vi "Increment Index.vi"(8 "error in (no error)":errorcluster, 11 "Abs_Waveform in":refnum<class "Abs_Waveform.lvclass">) -> (0 "error out":errorcluster, 3 "Abs_Waveform out":refnum<class "Abs_Waveform.lvclass">)   [LabVIEW 2021, in "Abs_Waveform.lvclass"]
uses:
  Abs_Waveform.lvclass
  Abs_Waveform.lvclass/Abs_Waveform.ctl
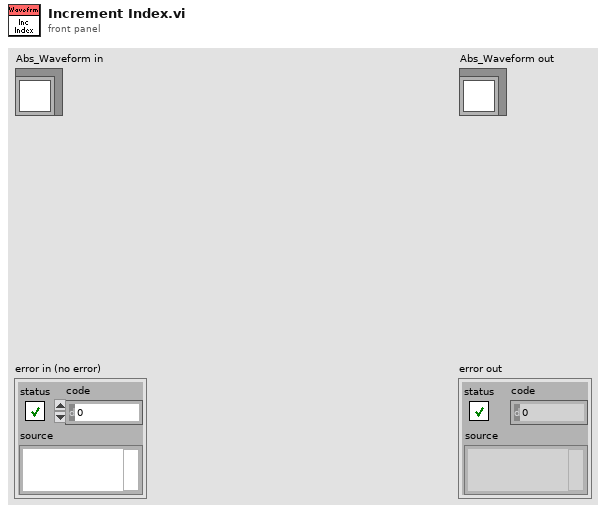
[diagram p1: front panel]
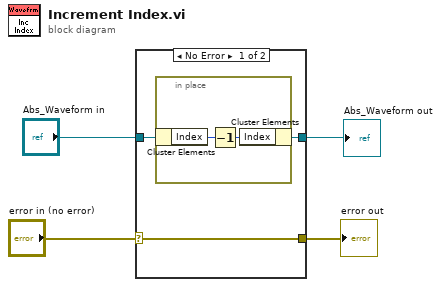
[diagram p0: block diagram]
diagram:
  n1 = case shown="No Error" "error in (no error)" {
    selector: "error in (no error)" -> [w5 w10]
    tunnel: "Abs_Waveform in" -> [w7 w11]
    tunnel: [w6 w11] -> w4
    tunnel: [w5 w10] -> w1
    frame No Error {
      n2 = in-place {
        n3 = in-place-cluster #1(w7) -> ("Index"=w9:i32)
        n4 = Decrement(x=w9) -> (x-1=w8:i32)
        n5 = in-place-cluster #1("Index"=w8) -> (w6:refnum<class "Abs_Waveform.lvclass">)
      }
    }
    frame Error {
    }
  }
  "error out" <- w1
  "Abs_Waveform out" <- w4
